vi "Convert Bytes to Number of BTI Records.vi"(11 "bytes read":i32) -> (3 "number of records read":i32)   [LabVIEW 2020, in "AIM ARINC 429 Engine.lvlib" / "Implementation.lvlib" / "Rx Execution Unit.lvclass"]
uses:
  Rx Execution Unit.lvclass
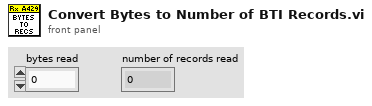
[diagram p1: front panel]
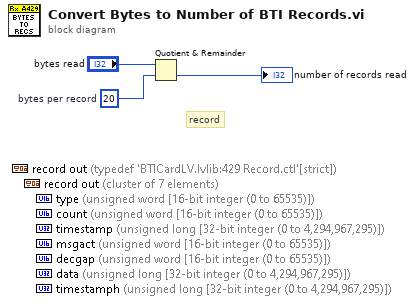
[diagram p0: block diagram]
diagram:
  w3 = 20  # bytes per record
  # "record"
  # "record"
  n1 = Quotient & Remainder(x="bytes read", y=w3) -> (floor(x/y)=→"number of records read":i32)  [unwired: 1 out]
